vi "DQFL2dll.vi"(8 "error in (no error)":errorcluster, 11 "Inputs":cluster{"d":dbl, "q":dbl, "z":dbl[], "kq":i32}={"d"=0.0, "q"=0.0, "z"=[0.0, 0.0, 0.0, 0.0, 0.0, 0.0, 0.0, 0.0, 0.0, 0.0, 0.0, 0.0, 0.0, 0.0, 0.0, 0.0, 0.0, 0.0, 0.0, 0.0], "kq"=0}) -> (0 "error out":errorcluster, 3 "Outputs":T1)   [LabVIEW 2021]
doc: "subroutine DQFL2 (d,q,z,kq,t,p,Dl,Dv,x,y,ierr,herr)\n\nflash calculation given bulk density, quality, and composition\n\nThis routine accepts only two-phase states as input; it is intended\nprimarily for use by the general density-quality flash routine\nDQFLSH. It may be called independently if the state is known to be\ntwo-phase. But beware--this routine does not check limits.\n\nINPUTS:\nd -- overall (bulk) molar density [mol/L]\nq -- vapor quality on a MOLAR basis [moles vapor/total moles]\nz -- overall (bulk) composition [array of mol frac]\nkq -- flag specifying units for input quality\n kq = 1 quality on MOLAR basis [moles vapor/total moles]\n kq = 2 quality on MASS basis [mass vapor/total mass]\n\nOUTPUTS:\nt -- temperature [K]\np -- pressure [kPa]\nDl -- molar density [mol/L] of the liquid phase\nDv -- molar density [mol/L] of the vapor phase\nx -- composition of liquid phase [array of mol frac]\ny -- composition of vapor phase [array of mol frac]\nierr -- error flag: 0 = successful\nherr -- error string (character*255 variable if ierr<>0)\nherr_length -- length of variable herr"
uses:
  REFPROP.dll
panel:
  # "REFPROP-DQFL2dll.vi"
  # "void  DQFL2dll(double *d, double *q, double *z, int32_t *kq, double *t, double *p, double *Dl, double *Dv, double *x, double *y, int32_t *ierr, CStr herr, int32_t *herr_length)"
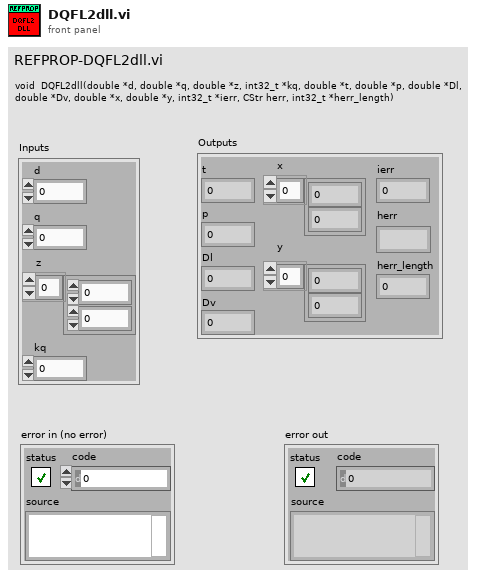
[diagram p1: front panel]
types:
  T1 = cluster{"t":dbl, "p":dbl, "Dl":dbl, "Dv":dbl, "x":dbl[], "y":dbl[], "ierr":i32, "herr":string, "herr_length":i32}
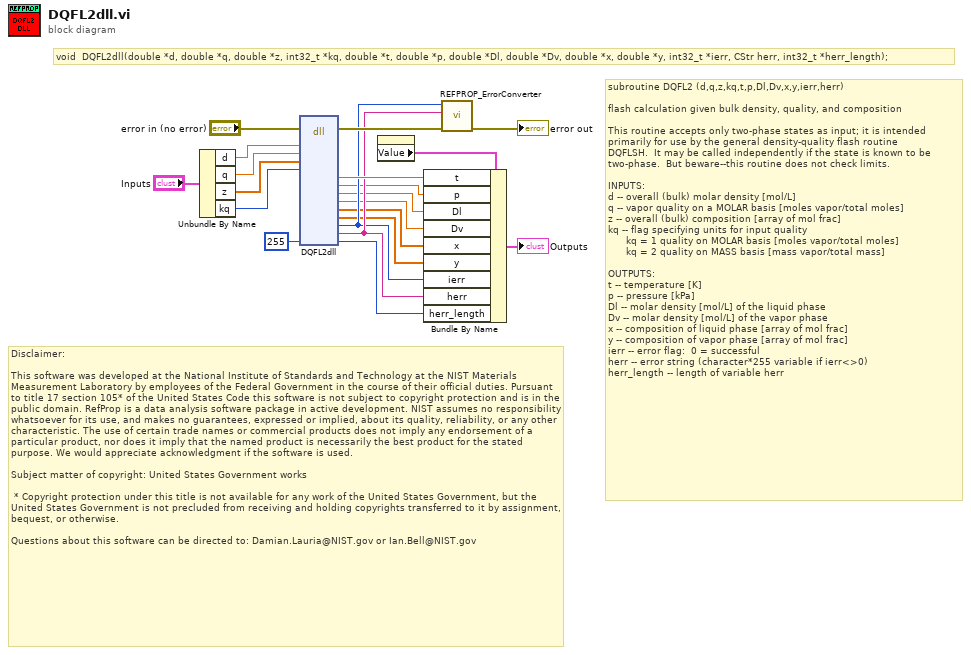
[diagram p0: block diagram]
diagram:
  # "Disclaimer:\n\nThis software was developed at the National Institute of Standards and Technology at the NIST Materials Measurement Laboratory by employees of the Federal Government in the course of their official duties. Pursuant to title 17 section 105* of the United States Code this software is not subject to copyright protection and is in the public domain. RefProp is a data analysis software package in active development. NIST assumes no responsibility whatsoever for its use, and makes no guarantees, expressed or implied, about its quality, reliability, or any other characteristic. The use of certain trade names or commercial products does not imply any endorsement of a particular product, nor does it imply that the named product is necessarily the best product for the stated purpose. We would appreciate acknowledgment if the software is used.\n \nSubject matter of copyright: United States Government works\n  \n * Copyright protection under this title is not available for any work of the United States Government, but the United States Government is not precluded from receiving and holding copyrights transferred to it by assignment, bequest, or otherwise.\n\nQuestions about this software can be directed to: Damian.Lauria@NIST.gov or Ian.Bell@NIST.gov"
  # "void  DQFL2dll(double *d, double *q, double *z, int32_t *kq, double *t, double *p, double *Dl, double *Dv, double *x, double *y, int32_t *ierr, CStr herr, int32_t *herr_length);"
  # "subroutine DQFL2 (d,q,z,kq,t,p,Dl,Dv,x,y,ierr,herr)\n\nflash calculation given bulk density, quality, and composition\n\nThis routine accepts only two-phase states as input; it is intended\nprimarily for use by the general density-quality flash routine\nDQFLSH.  It may be called independently if the state is known to be\ntwo-phase.  But beware--this routine does not check limits.\n\nINPUTS:\nd -- overall (bulk) molar density [mol/L]\nq -- vapor quality on a MOLAR basis [moles vapor/total moles]\nz -- overall (bulk) composition [array of mol frac]\nkq -- flag specifying units for input quality\n      kq = 1 quality on MOLAR basis [moles vapor/total moles]\n      kq = 2 quality on MASS basis [mass vapor/total mass]\n\nOUTPUTS:\nt -- temperature [K]\np -- pressure [kPa]\nDl -- molar density [mol/L] of the liquid phase\nDv -- molar density [mol/L] of the vapor phase\nx -- composition of liquid phase [array of mol frac]\ny -- composition of vapor phase [array of mol frac]\nierr -- error flag:  0 = successful\nherr -- error string (character*255 variable if ierr<>0)\nherr_length -- length of variable herr"
  n1 = Unbundle By Name("Inputs") -> ("d"=w15:dbl, "q"=w14:dbl, "z"=w13:dbl[], "kq"=w1:i32)
  n2 = dll-call lib="C:/Users/lauria/OneDrive - National Institute of Standards and Technology (NIST)/LabVIEW Projects/7 REFPROP/REFPROP-wrappers-master/REFPROP-wrappers-master/wrappers/Labview/REFPROP/REFPROP.*" fn="DQFL2dll"(error in="error in (no error)", "d"=w15, "q"=w14, "z"=w13, "kq"=w1, "herr_length"=255 ("ln")) -> (error out=w18:errorcluster, "t"=w10:dbl, "p"=w2:dbl, "Dl"=w3:dbl, "Dv"=w4:dbl, "x"=w5:dbl[], "y"=w6:dbl[], "ierr"=w7:i32, "herr"=w8:string, "herr_length"=w9:i32)  [unwired: 15 in, 1 out]
  n3 = property on="Outputs" class="Clust (strict)"() -> ("Value"=w12:T1)  [unwired: 2 in, 2 out]
  n4 = Bundle By Name(cluster=w12, "t"=w10, "p"=w2, "Dl"=w3, "Dv"=w4, "x"=w5, "y"=w6, "ierr"=w7, "herr"=w8, "herr_length"=w9) -> (→"Outputs":T1)
  n5 = call "REFPROP_ErrorConverter.vi"("error in (no error)"=w18, "Error Message"=w8, "Error Code"=w7) -> ("error out"=→"error out":errorcluster)  [unwired: 8 in]
